vi "Handle Messages.vi"(8 "error in (no error)":errorcluster, 9 "Message Data":variant, 10 "Message":string, 11 "Work Dispatcher In":refnum<class "Work Dispatcher.lvclass">) -> (0 "error out":errorcluster, 3 "Work Dispatcher Out":refnum<class "Work Dispatcher.lvclass">)   [LabVIEW 2020, in "Work Dispatcher.lvclass"]
uses:
  Work Dispatcher.lvclass
  C:/Program Files (x86)/National Instruments/LabVIEW 2020/vi.lib/Astemes/Triarc Framework/Helper Loop/Helper Loop.lvclass
  People/Process Job/Job Handler.lvclass
  Work Dispatcher.lvclass/Work Dispatcher.ctl
  <vilib>/Utility/error.llb/Error Cluster From Error Code.vi
  <vilib>/Astemes/Triarc Framework/Process/Public/Lifecycle/Get Lifecycle State.vi
  <vilib>/Astemes/Triarc Framework/Process/Process.lvclass
  <vilib>/Astemes/Triarc Framework/Helper Loop/Helper Loop.lvclass
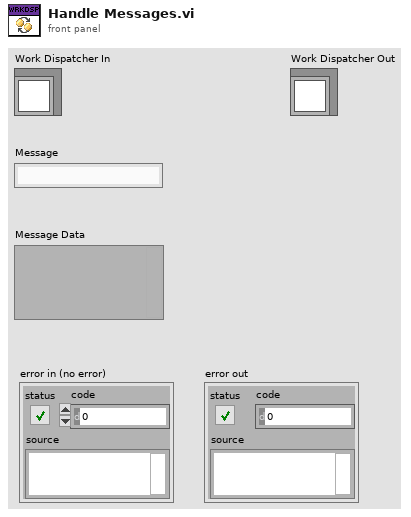
[diagram p1: front panel]
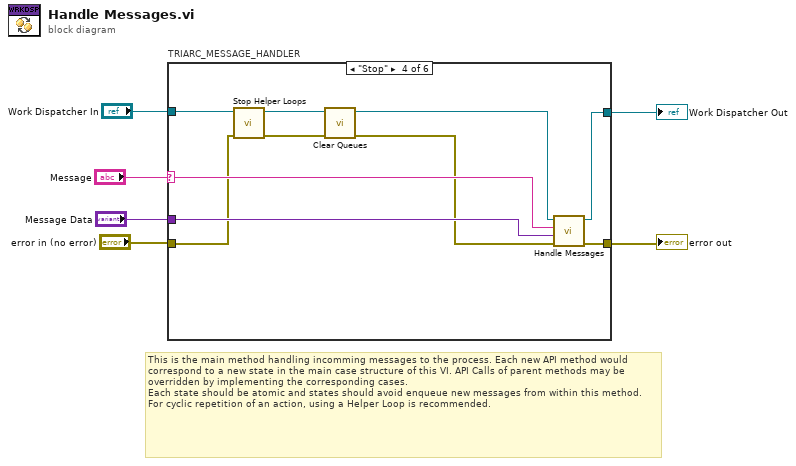
[diagram p0: block diagram]
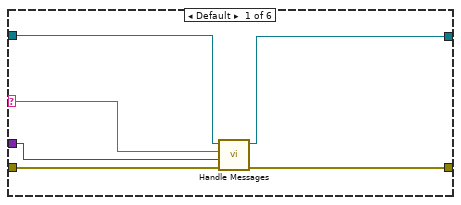
[diagram p2: hidden frame]
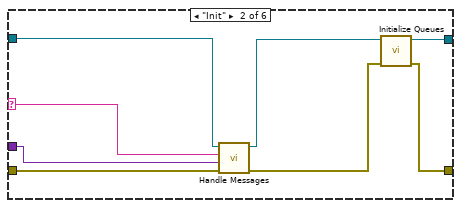
[diagram p3: hidden frame]
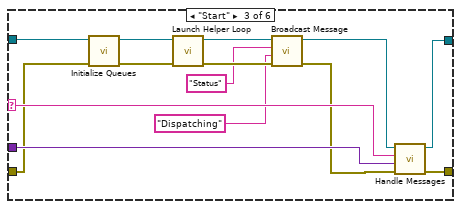
[diagram p4: hidden frame]
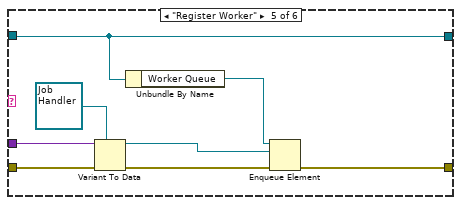
[diagram p5: hidden frame]
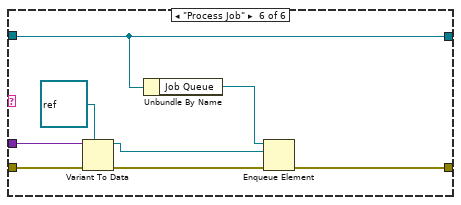
[diagram p6: hidden frame]
diagram:
  # "This is the main method handling incomming messages to the process. Each new API method would correspond to a new state in the main case structure of this VI. API Calls of parent methods may be overridden by implementing the corresponding cases.\nEach state should be atomic and states should avoid enqueue new messages from within this method. For cyclic repetition of an action, using a Helper Loop is recommended."
  n1 = case "TRIARC_MESSAGE_HANDLER" shown="\"Stop\"" "Message" {
    selector: "Message" -> [w10 w18 w32 w43 _ _]
    tunnel: "error in (no error)" -> [w9 w17 w31 w35 w52 w60]
    tunnel: "Work Dispatcher In" -> [w12 w20 w34 w39 w48 w55]
    tunnel: "Message Data" -> [w11 w19 w33 w44 w50 w57]
    tunnel: [w8 w13 w30 w42 w47 w56] -> w2
    tunnel: [w7 w15 w29 w41 w48 w55] -> w1
    frame Default {
      n2 = call-parent "Handle Messages.vi"("error in (no error)"=w9, "Message Data"=w11, "Message"=w10, "Process In"=w12) -> ("error out"=w8:errorcluster, "Process Out"=w7:refnum<class "Work Dispatcher.lvclass">)  [unwired: 6 in]
    }
    frame "Init" {
      n3 = call-parent "Handle Messages.vi"("error in (no error)"=w17, "Message Data"=w19, "Message"=w18, "Process In"=w20) -> ("error out"=w14:errorcluster, "Process Out"=w16:refnum<class "Work Dispatcher.lvclass">)  [unwired: 6 in]
      n4 = call "Initialize Queues.vi"("error in (no error)"=w14, "Work Dispatcher in"=w16) -> ("error out"=w13:errorcluster, "Work Dispatcher out"=w15:refnum<class "Work Dispatcher.lvclass">)  [unwired: 8 in]
    }
    frame "Start" {
      n5 = call "Initialize Queues.vi"("error in (no error)"=w31, "Work Dispatcher in"=w34) -> ("error out"=w28:errorcluster, "Work Dispatcher out"=w26:refnum<class "Work Dispatcher.lvclass">)  [unwired: 8 in]
      n6 = call <vilib>:"Launch Helper Loop.vi"("error in (no error)"=w28, "Helper Loop In"=w26) -> ("error out"=w27:errorcluster, "Helper Loop Out"=w24:refnum<class "Work Dispatcher.lvclass">)  [unwired: 8 in]
      n7 = call-dynamic "Broadcast Message.vi"("error in (no error)"=w27, "Message Data"="Dispatching" ("Message"), "Message"="Status", "Process In"=w24) -> ("error out"=w25:errorcluster, "Process Out"=w23:refnum<class "Work Dispatcher.lvclass">)  [unwired: 6 in]
      n8 = call-parent "Handle Messages.vi"("error in (no error)"=w25, "Message Data"=w33, "Message"=w32, "Process In"=w23) -> ("error out"=w30:errorcluster, "Process Out"=w29:refnum<class "Work Dispatcher.lvclass">)  [unwired: 6 in]
    }
    frame "Stop" {
      n9 = call <vilib>:"Stop Helper Loops.vi"("error in (no error)"=w35, "Helper Loop In"=w39) -> ("error out"=w36:errorcluster, "Helper Loop Out"=w37:refnum<class "Work Dispatcher.lvclass">)  [unwired: 8 in]
      n10 = call "Clear Queues.vi"("error in (no error)"=w36, "Work Dispatcher in"=w37) -> ("error out"=w40:errorcluster, "Work Dispatcher out"=w38:refnum<class "Work Dispatcher.lvclass">)  [unwired: 8 in]
      n11 = call-parent "Handle Messages.vi"("error in (no error)"=w40, "Message Data"=w44, "Message"=w43, "Process In"=w38) -> ("error out"=w42:errorcluster, "Process Out"=w41:refnum<class "Work Dispatcher.lvclass">)  [unwired: 6 in]
    }
    frame "Register Worker" {
      n12 = Variant To Data(error in=w52, type=refnum<class "Job Handler.lvclass"> refnum ("Process Job.lvclass"), Variant=w50) -> (data=w45:refnum<class "Job Handler.lvclass">, error out=w51:errorcluster)
      n13 = Unbundle By Name(w48) -> ("Worker Queue"=w46:refnum<queue>)
      n14 = Enqueue Element(queue=w46, element=w45, error in (no error)=w51) -> (error out=w47:errorcluster)  [unwired: 1 in, 2 out]
    }
    frame "Process Job" {
      n15 = Variant To Data(error in=w60, type=refnum<class> refnum ("LabVIEW Object"), Variant=w57) -> (data=w53:refnum<class>, error out=w59:errorcluster)
      n16 = Unbundle By Name(w55) -> ("Job Queue"=w54:refnum<queue>)
      n17 = Enqueue Element(queue=w54, element=w53, error in (no error)=w59) -> (error out=w56:errorcluster)  [unwired: 1 in, 2 out]
    }
  }
  "error out" <- w2
  "Work Dispatcher Out" <- w1
